vi "Fct_Limite_Température_v2.vi"(11 "Température":dbl) -> (2 "Booléen":bool, 3 "Chaîne":string)   [LabVIEW 2017]
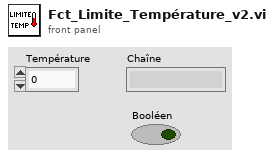
[diagram p1: front panel]
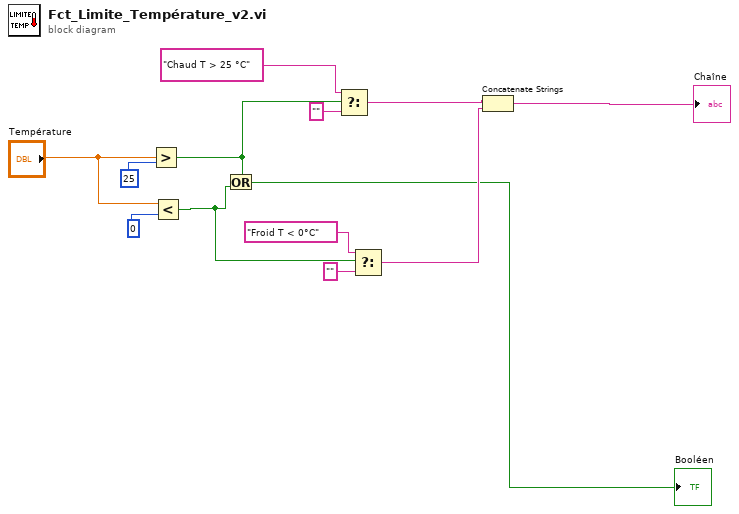
[diagram p0: block diagram]
diagram:
  n1 = Greater?(x="Température", y=25) -> (0:w5:bool)
  n2 = Less?(x="Température", y=0) -> (x < y?=w6:bool)
  n3 = Or(x=w5, y=w6) -> (x .or. y?=→"Booléen":bool)
  n4 = Select(t="Chaud T > 25 °C", s=w5, f="" ("cas faux")) -> (s? t:f=w11:string)
  n5 = Select(t="Froid T < 0°C", s=w6, f="" ("cas faux")) -> (s? t:f=w12:string)
  n6 = Concatenate Strings(w11, w12) -> (→"Chaîne":string)
